vi "mark_with_max_volume.vi"(1 "marksArray":T1[](array[typedef])) -> (0 "markValue":T1)   [LabVIEW 2015, in "PolyVIEW.lvclass"]
uses:
  PolyVIEW.lvclass
  actors/world/typedefs/markValue_cluster.ctl
  actors/world/typedefs/markValue.ctl
  actors/world/typedefs/markVolume.ctl
  actors/world/world.lvlib
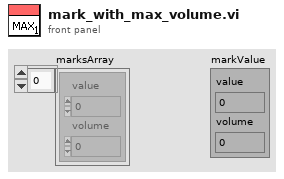
[diagram p1: front panel]
types:
  T1 = typedef "world.lvlib/markValue_cluster.ctl" = cluster{"value":T2, "volume":T3}
  T2 = typedef "world.lvlib/markValue.ctl" = u8
  T3 = typedef "world.lvlib/markVolume.ctl" = u16
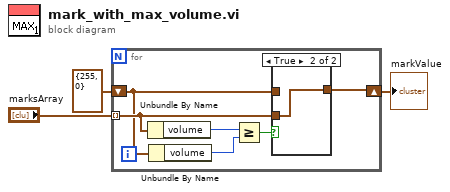
[diagram p0: block diagram]
diagram:
  n1 = for {
    tunnel: "marksArray" -> [w7] mode=indexing
    shift-right: [w6] -> w1
    shift-left: T1 {"value"=255, "volume"=0} ("markValue") -> [w5]
    n2 = Unbundle By Name(w7) -> ("volume"=w9:T3)
    n3 = Unbundle By Name(w5) -> ("volume"=w4:T3)
    n4 = Greater Or Equal?(x=w9, y=w4) -> (x >= y?=w8:bool)
    n5 = case shown="True" w8 {
      tunnel: w7 -> [_ w11]
      tunnel: [w10 w11] -> w6
      tunnel: w5 -> [w10 _]
      frame False {
      }
      frame True {
      }
    }
  }
  "markValue" <- w1
